vi "AWG Waveform Generator.vi"(0 "FGEN Resource Name":refnum<k15>, 5 "Transient":T1={"Delay - t1 (s)"=10.0, "Duration of the pulse (s)"=10.0, "Delay - t2 (s)"=10.0, "Load Current 1 - Iload1 (A)"=1.0, "Load Current 2 - Iload2 (A)"=0.0, "Slew rate A/us"=0.001, "Fgen Voltage to Current Ratio"=1.0} {"Fgen Voltage to Current Ratio" min=1.0 format="%#_6p"}, 7 "Offset (V)":dbl format="%#_13g", 11 "error in (no error)":errorcluster) -> (15 "error out":errorcluster)   [LabVIEW 2020, in "LDO Load Transient_AWG.lvlib"]
doc: "This example shows how to use the Arbitrary Waveform mode."
uses:
  LDO Load Transient_AWG.lvlib
  Typedefs/Transient Configuration.ctl
  <instrlib>/niFgen/niFgen.llb/niFgen Create Waveform (WDT).vi
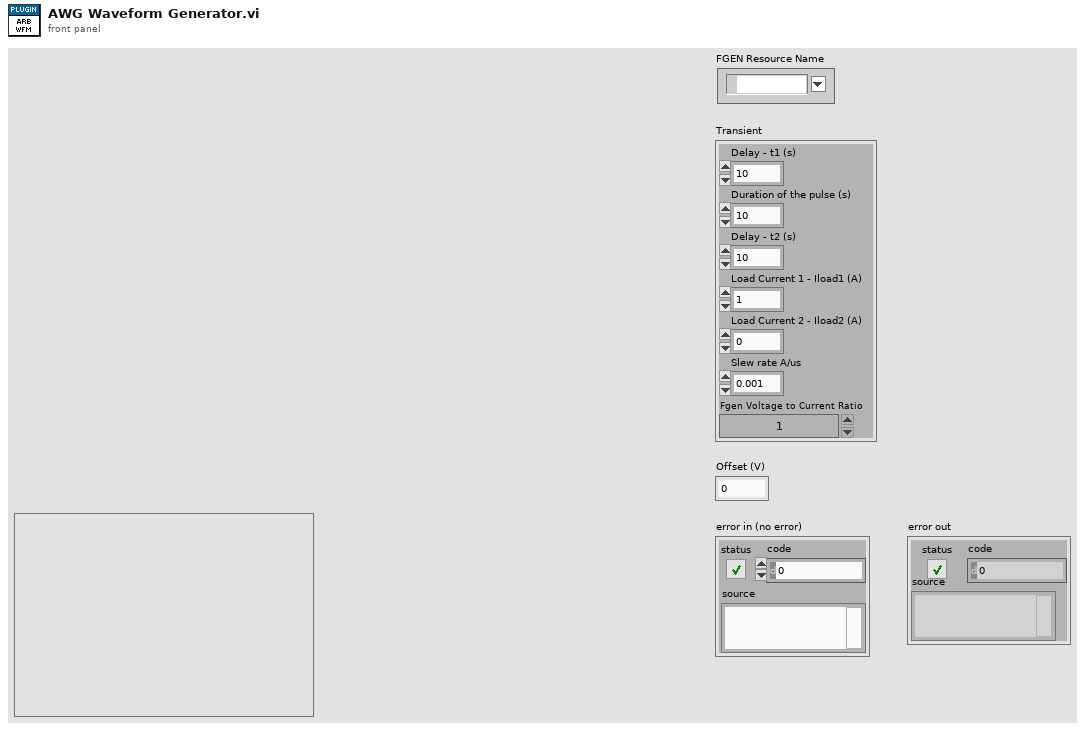
[diagram p1: front panel]
types:
  T1 = typedef "LDO Load Transient_AWG.lvlib/Transient Configuration.ctl" = cluster{"Delay - t1 (s)":dbl, "Duration of the pulse (s)":dbl, "Delay - t2 (s)":dbl, "Load Current 1 - Iload1 (A)":dbl, "Load Current 2 - Iload2 (A)":dbl, "Slew rate A/us":dbl, "Fgen Voltage to Current Ratio":dbl}
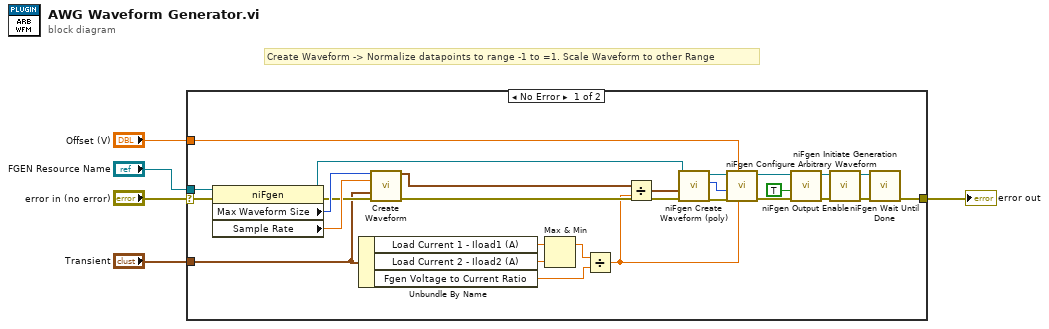
[diagram p0: block diagram]
diagram:
  # "Create Waveform -> Normalize datapoints to range -1 to =1. Scale Waveform to other Range"
  n1 = case shown="No Error" "error in (no error)" {
    selector: "error in (no error)" -> [w16 w33]
    tunnel: "FGEN Resource Name" -> [w32 _]
    tunnel: [w31 w33] -> w4
    tunnel: "Transient" -> [w12 _]
    tunnel: "Offset (V)" -> [w13 _]
    frame No Error {
      n2 = property class="niFgen"(reference=w32, error in=w16) -> (reference out=w19:refnum<k15>, error out=w20:errorcluster, "Max Waveform Size"=w22:i32, "Sample Rate"=w21:dbl)
      n3 = Unbundle By Name(w12) -> ("Load Current 1 - Iload1 (A)"=w11:dbl, "Load Current 2 - Iload2 (A)"=w10:dbl, "Fgen Voltage to Current Ratio"=w8:dbl)
      n4 = call "Create Waveform.vi"("Max Waveform Size"=w22, "Sample Rate"=w21, "Transient Configuration"=w12, "error in"=w20) -> ("Waveform Graph"=w14:waveform(dbl), "error out"=w15:errorcluster)  [unwired: 10 in]
      n5 = Max & Min(x=w11, y=w10) -> (max(x,y)=w9:dbl)  [unwired: 1 out]
      n6 = Divide(x=w9, y=w8) -> (x/y=w7:dbl)
      n7 = Divide(x=w14, y=w7) -> (x/y=w6:waveform(dbl))
      n8 = call-poly <instrlib>:"niFgen Create Waveform (poly).vi"("error in (no error)"=w15, "Waveform"=w6, "Instrument Handle"=w19) -> ("error out"=w29:errorcluster, "Waveform Handle"=w25:i32, "Instrument Handle Out"=w30:refnum<k15>)  [unwired: 6 in]
      n9 = call <instrlib>:"niFgen Configure Arbitrary Waveform.vi"("Gain"=w7, "Offset"=w13, "error in (no error)"=w29, "Waveform Handle"=w25, "Instrument Handle"=w30) -> ("error out"=w23:errorcluster, "Instrument Handle Out"=w24:refnum<k15>)  [unwired: 5 in]
      n10 = call <instrlib>:"niFgen Output Enable.vi"("error in (no error)"=w23, "Output Enable (default: True)"=TRUE ("output enable"), "Instrument Handle"=w24) -> ("error out"=w27:errorcluster, "Instrument Handle Out"=w28:refnum<k15>)  [unwired: 7 in]
      n11 = call <instrlib>:"niFgen Initiate Generation.vi"("error in (no error)"=w27, "Instrument Handle"=w28) -> ("error out"=w17:errorcluster, "Instrument Handle Out"=w18:refnum<k15>)  [unwired: 8 in]
      n12 = call <instrlib>:"niFgen Wait Until Done.vi"("error in (no error)"=w17, "Instrument Handle"=w18) -> ("error out"=w31:errorcluster)  [unwired: 8 in, 1 out]
    }
    frame Error {
    }
  }
  "error out" <- w4
